vi "Sample Out.vi"(8 "error in (no error)":errorcluster, 11 "Sample Line in":refnum<class "Sample Line.lvclass">) -> (0 "error out":errorcluster, 3 "Sample Line out":refnum<class "Sample Line.lvclass">)   [LabVIEW 2015, in "cRIO-Carbondioxide.lvlib" / "CO2-Actor.lvlib" / "Sample Line.lvclass"]
uses:
  Sample Line.lvclass
  CO2 Actor/CO2 Actor.lvclass
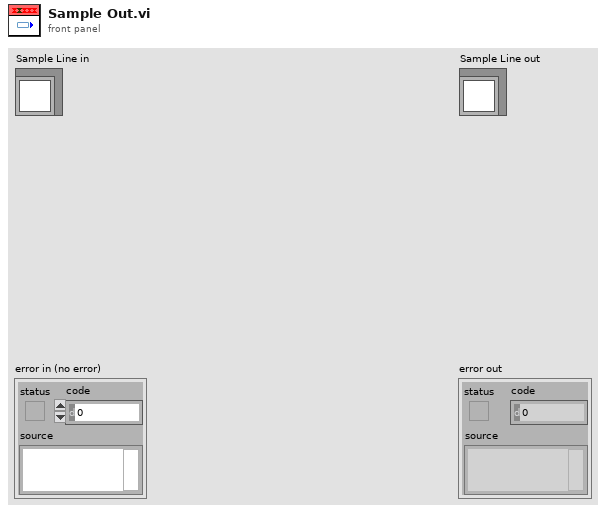
[diagram p1: front panel]
types:
  T1 = typedef "Sample Line State Enumerator.ctl" = enum16{"All lines closed", "Sample line 1.", "Sample line 2.", "Sample line 3.", "Sample line 4.", "Sample line 5.", "Out of range"}
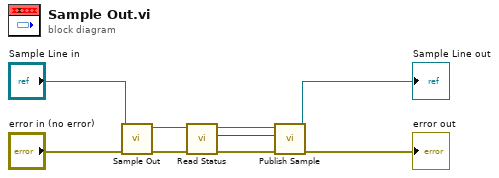
[diagram p0: block diagram]
diagram:
  n1 = call-parent "Sample Out.vi"("error in (no error)"="error in (no error)", "CO2 Actor in"="Sample Line in") -> ("error out"=w7:errorcluster, "CO2 Actor out"=w6:refnum<class "Sample Line.lvclass">)  [unwired: 8 in]
  n2 = call "Read Status.vi"("error in (no error)"=w7, "Sample Line in"=w6) -> ("error out"=w1:errorcluster, "Status"=w3:T1, "Sample Line out"=w2:refnum<class "Sample Line.lvclass">)  [unwired: 7 in]
  n3 = call "Publish Sample.vi"("error in (no error)"=w1, "Sample Line (All Closed)"=w3, "Sample Line in"=w2) -> ("error out"=→"error out":errorcluster, "Sample Line in 2"=→"Sample Line out":refnum<class "Sample Line.lvclass">)  [unwired: 7 in]
